vi "Is Class Not Interface Without Loading.vi"(9 "path":path, 10 "delimited name":string, 11 "type":T1) -> (3 "is class":bool)   [LabVIEW 2020]
uses:
  <vilib>/Utility/lvfile.llb/LVFileType.ctl
  <vilib>/Utility/lvfile.llb/NI_FileType.lvlib
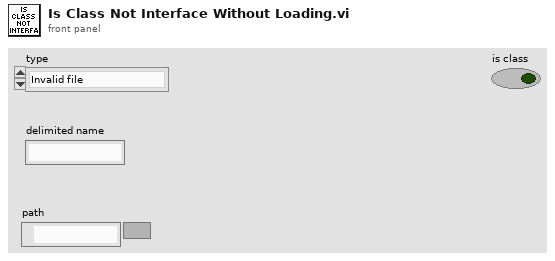
[diagram p1: front panel]
types:
  T1 = typedef "NI_FileType.lvlib/LVFileType.ctl" = enum32{"Invalid file", "Unknown type", "Instrument", "Control", "Polymorphic VI", "Project", "Library", "LVClass", "XControl", "XNode", "Shared library", ".NET assembly", "ActiveX interface", "CIN", "Run-time menu", "Palette menu", "Help file", "LLB", "XNode Edit Dependency", "Class Private Data Control", "Statechart", "MathScript .m file", "Ladder Diagram", "LVLibp", "XNode Build Dependency"}
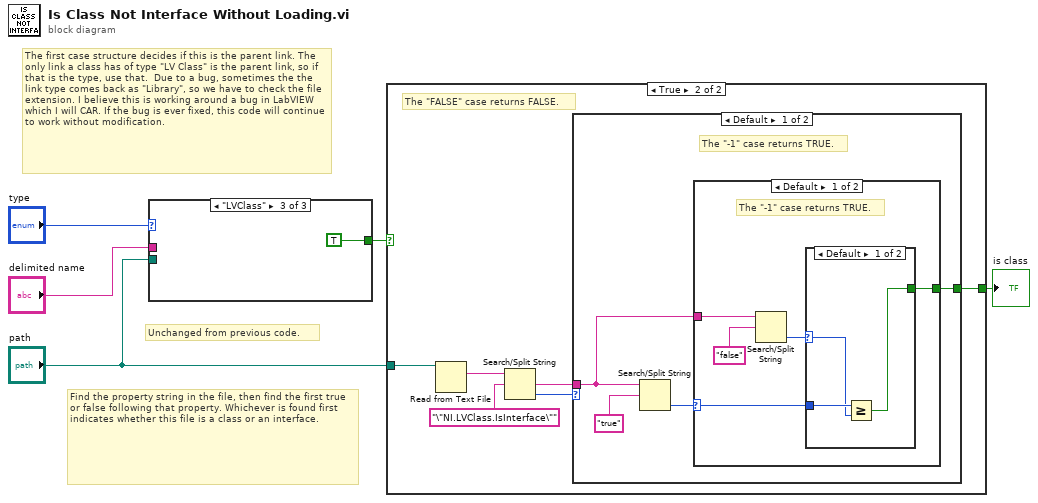
[diagram p0: block diagram]
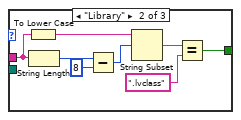
[diagram p3: hidden frame]
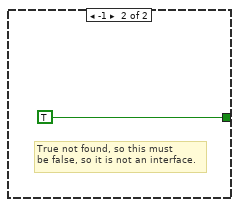
[diagram p6: hidden frame]
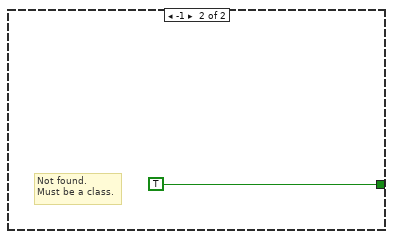
[diagram p7: hidden frame]
diagram:
  # "Find the property string in the file, then find the first true or false following that property. Whichever is found first indicates whether this file is a class or an interface."
  # "Unchanged from previous code."
  # "The first case structure decides if this is the parent link. The only link a class has of type \"LV Class\" is the parent link, so if that is the type, use that.  Due to a bug, sometimes the the link type comes back as \"Library\", so we have to check the file extension. I believe this is working around a bug in LabVIEW which I will CAR. If the bug is ever fixed, this code will continue to work without modification."
  n1 = case shown="\"LVClass\"" "type" {
    tunnel: "delimited name" -> [_ w10 _]
    tunnel: [_ w7 TRUE] -> w3
    tunnel: "path" -> [_ _ _]
    frame Default {
    }
    frame "Library" {
      n2 = To Lower Case(string=w10) -> (all lower case string=w6:string)
      n3 = String Length(string=w10) -> (length=w13:i32)
      n4 = Subtract(x=w13, y=8) -> (x-y=w11:i32)
      n5 = String Subset(string=w6, offset (0)=w11) -> (substring=w9:string)  [unwired: 1 in]
      n6 = Equal?(x=w9, y=".lvclass") -> (x = y?=w7:bool)
    }
    frame "LVClass" {
    }
  }
  n7 = case shown="True" w3 {
    selector: w3 -> [w15 _]
    tunnel: [w15 w20] -> w2
    tunnel: "path" -> [_ w21]
    frame False {
    }
    frame True {
      # "The \"FALSE\" case returns FALSE."
      n8 = Read from Text File(file (use dialog)=w21) -> (text=w19:string)  [unwired: 3 in, 3 out]
      n9 = Search/Split String(string=w19, search string/char (-)="\"NI.LVClass.IsInterface\"" ("y")) -> (match + rest of string=w16:string, offset of match=w17:i32)  [unwired: 1 in, 1 out]
      n10 = case shown="Default" w17 {
        tunnel: [w23 TRUE] -> w20
        tunnel: w16 -> [w22 _]
        frame Default {
          # "The \"-1\" case returns TRUE."
          n11 = Search/Split String(string=w22, search string/char (-)="true" ("y")) -> (offset of match=w24:i32)  [unwired: 1 in, 2 out]
          n12 = case shown="Default" w24 {
            selector: w24 -> [w26 _]
            tunnel: [w27 TRUE] -> w23
            tunnel: w22 -> [w29 _]
            frame Default {
              # "The \"-1\" case returns TRUE."
              n13 = Search/Split String(string=w29, search string/char (-)="false" ("y")) -> (offset of match=w28:i32)  [unwired: 1 in, 2 out]
              n14 = case shown="Default" w28 {
                selector: w28 -> [w32 _]
                tunnel: [w31 _] -> w27
                tunnel: w26 -> [w33 _]
                frame Default {
                  n15 = Greater Or Equal?(x=w33, y=w32) -> (x >= y?=w31:bool)
                }
                frame -1 {
                  # "Must be true,\nso this is an\ninterface."
                }
              }
            }
            frame -1 {
              # "True not found, so this must\nbe false, so it is not an interface."
            }
          }
        }
        frame -1 {
          # "Not found.\nMust be a class."
        }
      }
    }
  }
  "is class" <- w2
